vi "2_03.vi"() -> ()   [LabVIEW 2018]
uses:
  <vilib>/measure/macond.llb/Continuous Waveform Convolution for 1 Chan.vi
  <vilib>/measure/NI_MAPro.lvlib
  <vilib>/measure/NI_MABase.lvlib
  <vilib>/Analysis/NI_AALBase.lvlib
panel:
  out "Waveform Graph":dbl[](graph)
  in  "N":dbl
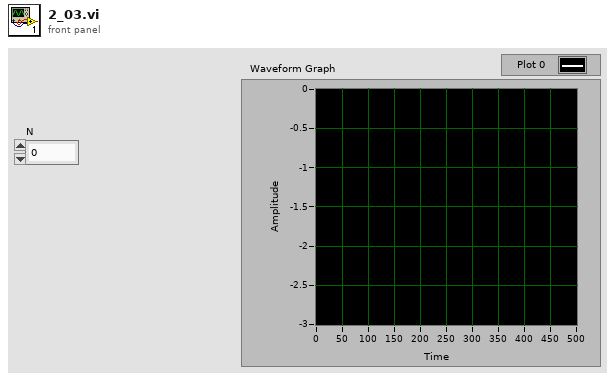
[diagram p1: front panel]
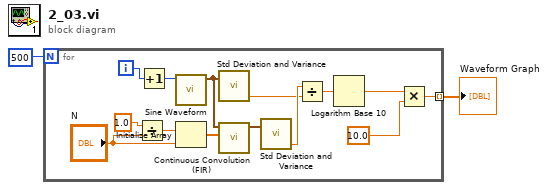
[diagram p0: block diagram]
diagram:
  n1 = for {
    N: 500 -> [_]
    tunnel: [w4] -> w1 mode=indexing
    i -> [w13]
    n2 = Divide(x=1.0, y="N") -> (x/y=w15:dbl)
    n3 = Increment(x=w13) -> (x+1=w12:i32)
    n4 = call <vilib>:"Sine Waveform.vi"("frequency"=w12) -> ("signal out"=w3:waveform(dbl))  [unwired: 9 in, 1 out]
    n5 = Initialize Array(w15, "N") -> (w10:dbl[])
    n6 = call <vilib>:"Std Deviation and Variance.vi"("X"=w3) -> ("variance"=w8:dbl)  [unwired: 1 in, 2 out]
    n7 = call-poly <vilib>:"Continuous Convolution (FIR).vi"("kernel"=w10, "signal in"=w3) -> ("signal out"=w11:waveform(dbl))  [unwired: 8 in, 1 out]
    n8 = call <vilib>:"Std Deviation and Variance.vi"("X"=w11) -> ("variance"=w9:dbl)  [unwired: 1 in, 2 out]
    n9 = Divide(x=w9, y=w8) -> (x/y=w7:dbl)
    n10 = Logarithm Base 10(1:w7) -> (0:w6:dbl)
    n11 = Multiply(x=w6, y=10.0) -> (x*y=w4:dbl)
  }
  "Waveform Graph" <- w1
